vi "tempMeasuringDevice.vi"() -> ()   [LabVIEW 2017]
panel:
  in  "?":bool
  in  "increase timer with (s)":dbl=3600.0 format="%#_13g"
  in  "iterate in (ms)":u32
  in  "file path":path
  in  "Start date":timestamp=timestamp(2713996800 s since 1904-01-01) format="%<%X\n%x>T"
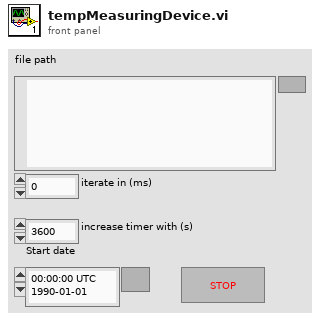
[diagram p1: front panel]
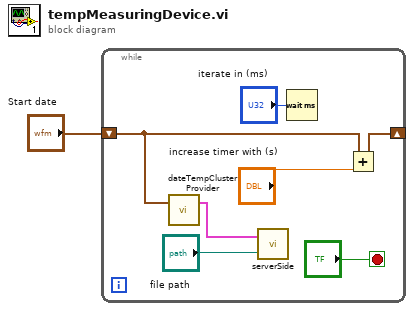
[diagram p0: block diagram]
diagram:
  n1 = while {
    shift-right: [w7] -> _
    shift-left: "Start date" -> [w3]
    stop <- "?" stop-if-true
    n2 = call "dateTempClusterProvider.vi"("Time Stamp"=w3) -> ("Cluster"=w2:cluster{"Time Stamp":timestamp, "Numeric":i32})  [unwired: 2 in]
    n3 = call "serverSide.vi"("file path (use dialog)"="file path", "Cluster"=w2) -> ()  [unwired: 1 in]
    n4 = Wait (ms)(milliseconds to wait="iterate in (ms)") -> ()  [unwired: 1 out]
    n5 = Add(x=w3, y="increase timer with (s)") -> (x+y=w7:timestamp)
  }
